vi "FTW-TestStep-Template-Core_Initialize.vi"(0 "Initialization Sequence":string, 5 "FTW Actor Instance Configuration":string, 11 "error in (no error)":errorcluster) -> (4 "FTW-TestStep-Template-Core Out":refnum<class "FTW-TestStep-Template-Core.lvclass">, 6 "Event Refnums":T1, 10 "Refresh Period":dbl, 15 "error out":errorcluster)   [LabVIEW 2015, in "FTW-TestStep-Template-Core.lvclass"]
uses:
  FTW-TestStep-Template-Core.lvclass
  source/actor/Message/Request/FTW-Message-IncomingRequest.lvclass
  source/actor/Message/Base/FTW-Message.lvclass
  FTW-TestStep-Template-Core.lvclass/FTW-TestStep-Template-Core.ctl
  source/JSON/core/FTW-JSON-Core-EncodingFlags.vi
  source/JSON/FTW-JSON-Parse.vi
  source/Reflection/FTW-Reflection-Type.vi
  source/CodeGen/JSON Deserialize/FTW-JSON-Core-GetFlattenedValue.vi
  source/CodeGen/JSON Deserialize/FTW-JSON-Deserialize.xnode
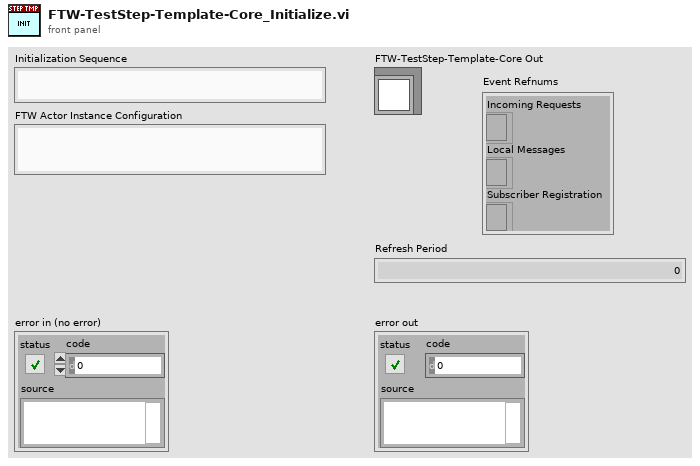
[diagram p1: front panel]
types:
  T1 = cluster{"Incoming Requests":refnum<event-registration>, "Local Messages":refnum<event-registration>, "Subscriber Registration":refnum<event-registration>}
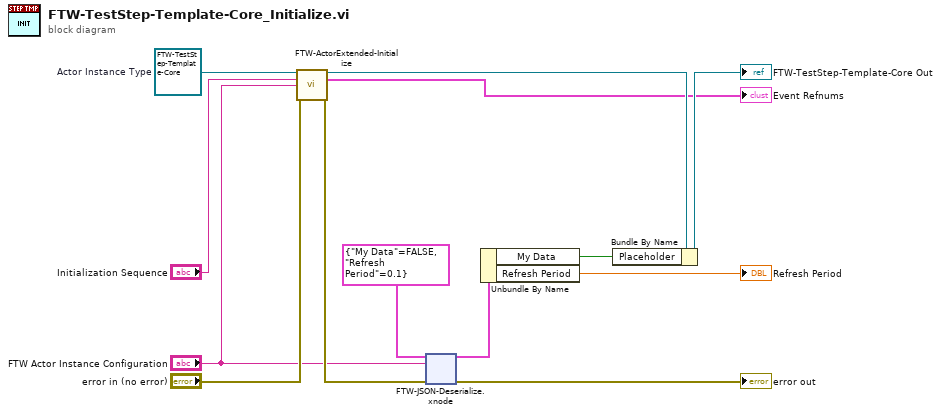
[diagram p0: block diagram]
diagram:
  w13 = refnum<class "FTW-TestStep-Template-Core.lvclass"> refnum  # Actor Instance Type
  n1 = call-dynamic "FTW-ActorExtended-Initialize.vi"("FTW Actor Instance Type"=w13, "Initialization Job Sequence"="Initialization Sequence", "Actor Instance Configuration"="FTW Actor Instance Configuration", "error in"="error in (no error)") -> ("FTW Actor Instance"=w7:refnum<class "FTW-TestStep-Template-Core.lvclass">, "Event Refnums"=→"Event Refnums":T1, "error out"=w5:errorcluster)  [unwired: 9 in]
  n2 = xnode "FTW-JSON-Deserialize.xnode"("Type and Defaults"=cluster{"My Data":bool, "Refresh Period":dbl} {"My Data"=FALSE, "Refresh Period"=0.1}, "JSON String"="FTW Actor Instance Configuration", "error in"=w5) -> ("Values"=w9:cluster{"My Data":bool, "Refresh Period":dbl}, "error out"=→"error out":errorcluster)
  n3 = Unbundle By Name(w9) -> ("My Data"=w8:bool, "Refresh Period"=→"Refresh Period":dbl)
  n4 = Bundle By Name(cluster=w7, "Placeholder"=w8) -> (→"FTW-TestStep-Template-Core Out":refnum<class "FTW-TestStep-Template-Core.lvclass">)
